vi "AlighnAndResample.vi"(7 "Resample to longest dt (F:Resample to shortest dt)":bool, 8 "error in (no error)":errorcluster, 11 "waveforms in":waveform(dbl)[](array[waveform])) -> (0 "error out":errorcluster, 3 "waveforms out":waveform(dbl)[](array[waveform]))   [LabVIEW 2015]
uses:
  Instance           1 25Saved   AlighnAndResample .vi
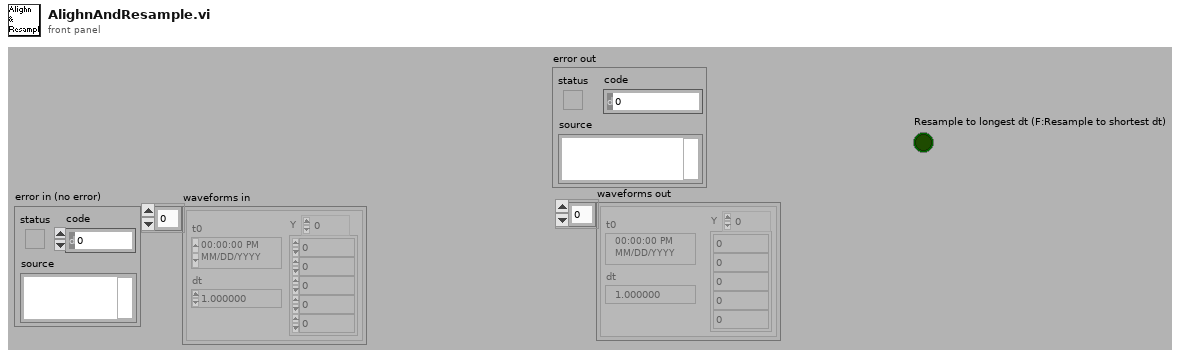
[diagram p1: front panel]
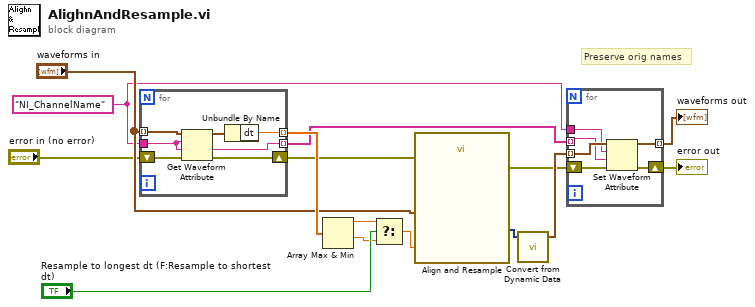
[diagram p0: block diagram]
diagram:
  w2 = "NI_ChannelName" ("name")
  # "Preserve orig names"
  n1 = for {
    tunnel: "waveforms in" -> [w21] mode=indexing
    tunnel: [w22] -> w15 mode=indexing
    shift-right: [w19] -> w5
    shift-left: "error in (no error)" -> [w17]
    tunnel: w2 -> [w16]
    tunnel: [w18] -> w1 mode=indexing
    n2 = Get Waveform Attribute(4:w17, 5:w16, 6:w16, 7:w21) -> (0:w19:errorcluster, 1:w18:string, 3:w20:waveform(dbl))  [unwired: 1 out]
    n3 = Unbundle By Name(w20) -> ("dt"=w22:dbl)
  }
  n4 = Array Max & Min(array=w15) -> (max value=w12:dbl, min value=w11:dbl)  [unwired: 2 out]
  n5 = Select(t=w12, s="Resample to longest dt (F:Resample to shortest dt)", f=w11) -> (s? t:f=w10:dbl)
  n6 = call "Align and Resample"("dt"=w10, "error in (no error)"=w5, "Signals"="waveforms in") -> ("error out"=w4:errorcluster, "Resampled Signals"=w8:dynamicdata)  [unwired: 1 in, 6 out]
  n7 = call "Convert from Dynamic Data"("Dynamic Data Type"=w8) -> ("Array of Waveform"=w7:waveform(dbl)[])  [unwired: 3 in]
  n8 = for {
    tunnel: [w28] -> w9 mode=indexing
    tunnel: w7 -> [w27] mode=indexing
    shift-right: [w25] -> w3
    shift-left: w4 -> [w26]
    tunnel: w2 -> [w24]
    tunnel: w1 -> [w23] mode=indexing
    n9 = Set Waveform Attribute(4:w26, 5:w23, 6:w24, 7:w27) -> (0:w25:errorcluster, 3:w28:waveform(dbl))  [unwired: 1 out]
  }
  "error out" <- w3
  "waveforms out" <- w9
